vi "Get TMOD.vi"(8 "error in":errorcluster, 11 "SR 3XX HVPS in":refnum<class "SR 3XX HVPS.lvclass">) -> (0 "error out":errorcluster, 2 "Trip Mode":T1, 3 "SR 3XX HVPS out":refnum<class "SR 3XX HVPS.lvclass">)   [LabVIEW 2013, in "SR 3XX HVPS.lvclass"]
doc: "Retrieve the current trip reset mode: manual or auto."
uses:
  SR 3XX HVPS.lvclass
  Control/Trip Mode.ctl
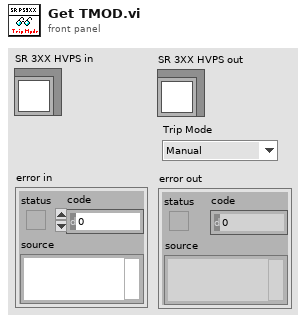
[diagram p1: front panel]
types:
  T1 = typedef "Trip Mode.ctl" = enum8{"Manual", "Auto"}
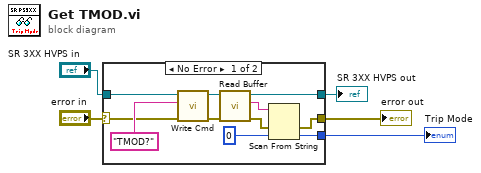
[diagram p0: block diagram]
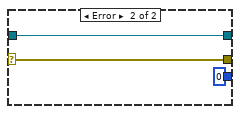
[diagram p2: hidden frame]
diagram:
  n1 = case shown="No Error" "error in" {
    selector: "error in" -> [w12 w19]
    tunnel: [w8 w19] -> w4
    tunnel: [w11 w18] -> w2
    tunnel: "SR 3XX HVPS in" -> [w16 w18]
    tunnel: [w6 u8 0] -> w1
    frame No Error {
      n2 = call "Write Cmd.vi"("error in"=w12, "Cmd"="TMOD?", "SR 3XX HVPS in"=w16) -> ("error out"=w13:errorcluster, "SR 3XX HVPS out"=w14:refnum<class "SR 3XX HVPS.lvclass">)  [unwired: 7 in]
      n3 = call "Read Buffer.vi"("error in"=w13, "SR 3XX HVPS in"=w14) -> ("error out"=w9:errorcluster, "ReadData"=w10:string, "SR 3XX HVPS out"=w11:refnum<class "SR 3XX HVPS.lvclass">)  [unwired: 7 in]
      n4 = Scan From String(input string=w10, error in=w9, default 1=u8 0) -> (error out=w8:errorcluster, output 1=w6:u8)  [unwired: 2 in, 2 out]
    }
    frame Error {
    }
  }
  "error out" <- w4
  "SR 3XX HVPS out" <- w2
  "Trip Mode" <- w1
